vi "Set Wheel Property by Name.vi"(7 "wheel indexes":i32[](array[numeric]), 8 "error in (no error)":errorcluster, 9 "parameter value":variant, 10 "parameter name":string, 11 "steering frame reference in":refnum<data-value>) -> (0 "error out":errorcluster, 3 "steering frame reference out":refnum<data-value>)   [LabVIEW 2017, in "NI_Robotics_Configure Steering Frame.lvlib"]
uses:
  <vilib>/robotics/Dialog/Configure Steering Frame/NI_Robotics_Configure Steering Frame.lvlib
  <vilib>/robotics/Steering/Steering Frame/NI_Robotics_Steering Frame.lvclass
  <vilib>/robotics/Steering/Steering Frame/NI_Robotics_Steering Frame.lvclass/NI_Robotics_Steering Frame.ctl
  <vilib>/robotics/Steering/Steering Frame/Get Multiple Wheels in Steering Frame.vi
  <vilib>/robotics/Steering/Wheel/NI_Robotics_Wheel.lvclass
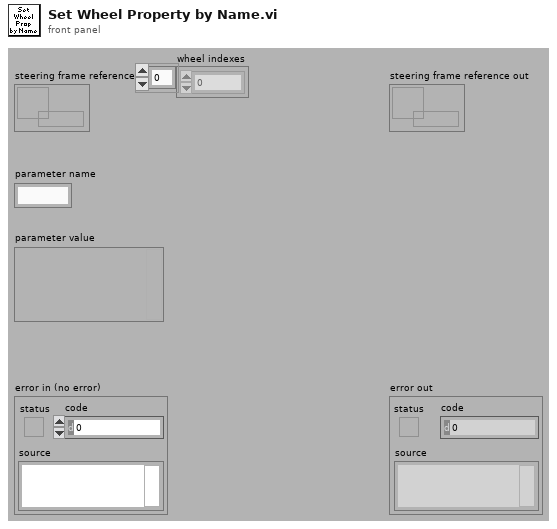
[diagram p1: front panel]
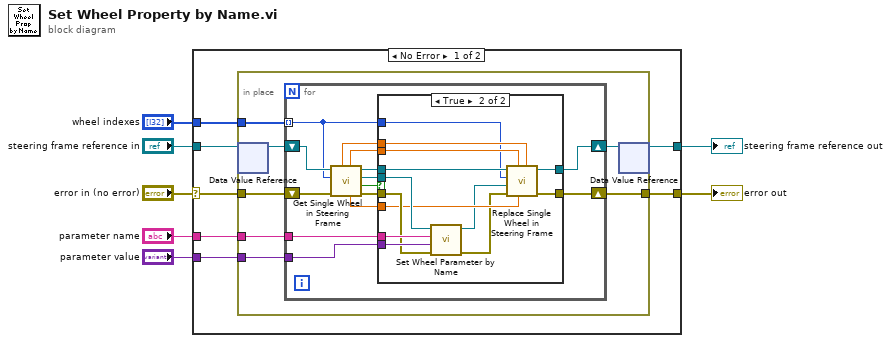
[diagram p0: block diagram]
diagram:
  n1 = case shown="No Error" "error in (no error)" {
    selector: "error in (no error)" -> [w10 w52]
    tunnel: [w9 w52] -> w6
    tunnel: "steering frame reference in" -> [w14 w51]
    tunnel: [w13 w51] -> w4
    tunnel: "wheel indexes" -> [w8 _]
    tunnel: "parameter name" -> [w12 _]
    tunnel: "parameter value" -> [w11 _]
    frame No Error {
      n2 = in-place {
        in-place-border: w8 -> [w17]
        in-place-border: w12 -> [w21]
        in-place-border: w11 -> [w20]
        in-place-border: w10 -> [w18]
        in-place-border: [w15] -> w9
        n3 = in-place-dvr #1(w14) -> (w19:refnum<class "NI_Robotics_Steering Frame.lvclass">)  [unwired: 1 out]
        n4 = for {
          tunnel: w21 -> [w35]
          tunnel: w20 -> [w34]
          tunnel: w17 -> [w25] mode=indexing
          shift-right: [w24] -> w16
          shift-left: w19 -> [w33]
          shift-right: [w23] -> w15
          shift-left: w18 -> [w30]
          n5 = call <vilib>:"Get Single Wheel in Steering Frame.vi"("error in (no error)"=w30, "wheel index"=w25, "steering frame in"=w33) -> ("error out"=w31:errorcluster, "found?"=w22:bool, "wheel"=w32:refnum<class "NI_Robotics_Wheel.lvclass">, "steering frame out"=w29:refnum<class "NI_Robotics_Steering Frame.lvclass">, "frame angle (rad)"=w26:dbl, "y position"=w28:dbl, "x position"=w27:dbl)  [unwired: 2 in]
          n6 = case shown="True" w22 {
            tunnel: w35 -> [_ w50]
            tunnel: w34 -> [_ w49]
            tunnel: w32 -> [_ w48]
            tunnel: w31 -> [w36 w47]
            tunnel: w29 -> [w37 w46]
            tunnel: w28 -> [_ w45]
            tunnel: w27 -> [_ w44]
            tunnel: w26 -> [_ w43]
            tunnel: w25 -> [_ w41]
            tunnel: [w37 w39] -> w24
            tunnel: [w36 w38] -> w23
            frame False {
            }
            frame True {
              n7 = call-dynamic "Set Wheel Parameter by Name.vi"("error in (no error)"=w47, "parameter value"=w49, "parameter name"=w50, "wheel in"=w48) -> ("error out"=w40:errorcluster, "wheel out"=w42:refnum<class "NI_Robotics_Wheel.lvclass">)  [unwired: 5 in, 1 out]
              n8 = call <vilib>:"Replace Single Wheel in Steering Frame.vi"("x position"=w44, "frame angle (rad)"=w43, "y position"=w45, "error in (no error)"=w40, "wheel"=w42, "wheel index"=w41, "steering frame in"=w46) -> ("error out"=w38:errorcluster, "steering frame out"=w39:refnum<class "NI_Robotics_Steering Frame.lvclass">)  [unwired: 2 in, 1 out]
            }
          }
        }
        n9 = in-place-dvr #1(w16) -> (w13:refnum<data-value>)  [unwired: 1 out]
      }
    }
    frame Error {
    }
  }
  "error out" <- w6
  "steering frame reference out" <- w4
